vi "Cache User Parameters_minimal_test.vi"(8 "error in (no error)":errorcluster, 11 "SHIFTER DATA in":T1) -> (0 "error out":errorcluster, 3 "SHIFTER DATA out":T1)   [LabVIEW 2013, in "main.lvlib"]
uses:
  Components/TypeDef - SHIFTER.ctl
  Components/Dependencies.llb/Exit Event Ref.ctl
  New Design/Controls/Reference Cluster.ctl
  Controls/Enum Variables.ctl
  main.lvlib
  Components/Dependencies.llb/TLB_Dependencies.lvlib
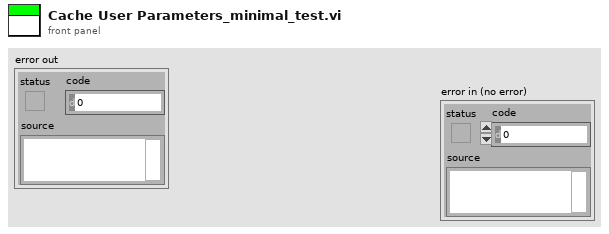
[diagram p1: front panel]
types:
  T1 = typedef "main.lvlib/TypeDef - SHIFTER.ctl" = cluster{"Exit Event":T2, "Terminate Error":errorcluster, "User Parameter Controls":refnum<vi>[], "User Parameters":cluster{"Name":string, "CPR Number":string, "Measuring Type ":string, "Measuring Technique":string, "Measuring Limb":string, "Operator":string, "Doctor":string, "Comment":string, "AdditionalInfo":string, "RightArm":string[][], "LeftArm":string[][], "PalpationRight":string, "PalpationLeft":string, "Puls":dbl, "Temp One":dbl, "Temp Two":dbl, "ActivityBox":bool}, "System Parameters":cluster{"Paper Running?":bool, "GraphSelection":bool, "Date":string, "Active Page":string}, "Data Acquisition":cluster{"Acquisition":bool, "DAQmx Task":refnum<k21>, "DAQmx Error":errorcluster, "Record number":dbl, "RecordPath":path, "AcqDataRef":refnum<vi>, "Duration":timestamp, "Queue":refnum<queue>, "Control?":bool, "RelativeRecordPath":path}, "Reference signal":cluster{"DAQmx  Task ":refnum<k21>, "Monitor":bool, "Events":dbl, "Time":timestamp, "NullEvents":dbl, "RefDataRef":refnum<vi>, "Queue":refnum<queue>}, "Data Process":cluster{"SubpanelRef":refnum<vi>, "ActiveItemTag":string, "Queue":refnum<queue>}, "System Parameter Controls":refnum<vi>[], "Database":cluster{"PatientdataRef":refnum<file>, "PatientdataPath":path, "Blue Pressure":dbl, "Red Pressure":dbl, "ActiveItemTag":string, "Height Adjustment":dbl, "BluePositionArray":dbl[][], "RedPositionArray":dbl[][], "JournalPath":path}, "MWL":cluster{"PatientID":string, "Name":string, "DICOM Info":path, "DICOM Variables":string[], "Worklist":string[][]}, "Control":cluster{"Queue":refnum<queue>, "SignalCluster":cluster{"Pump":bool, "Finger":bool, "Ankle":bool, "Fast Def":bool, "Slow Def":bool, "Init Cal":bool, "Table Pres":bool, "Table":bool}}, "PageMenu":cluster{"VI Reference":refnum<vi>, "Queue":refnum<queue>}, "Profile":cluster{"VI Reference":refnum<vi>, "Queue":refnum<queue>}, "Configuration":cluster{"VI Reference":refnum<vi>, "Queue":refnum<queue>}, "Acquisition":cluster{"VI Reference":refnum<vi>, "Queue":refnum<queue>}, "Data":cluster{"VI Reference":refnum<vi>, "Queue":refnum<queue>}, "Journal":cluster{"VI Reference":refnum<vi>, "Queue":refnum<queue>}, "cRef":T3, "Bluetooth":cluster{"Queue":refnum<queue>, "VI Reference":refnum<vi>}}
  T2 = typedef "main.lvlib/TLB_Dependencies.lvlib/Exit Event Ref.ctl" = refnum<user-event>
  T3 = typedef "main.lvlib/Reference Cluster.ctl" = cluster{"Menu":cluster{"References":cluster{"Stop Acq":refnum<vi>, "MenuExit":refnum<vi>, "MenuStartADC":refnum<vi>, "PersonalInfoString":refnum<vi>, "Profile":refnum<vi>, "Configuration":refnum<vi>, "Acquisition":refnum<vi>, "Data":refnum<vi>, "Journal":refnum<vi>}}, "Profile":cluster{"References":cluster{"Search Patient ID":refnum<vi>, "Name":refnum<vi>, "CommentStr":refnum<vi>, "Listbox Patient ID":refnum<vi>, "ListboxDoctor":refnum<vi>, "ListboxOperator":refnum<vi>, "HospitalName":refnum<vi>, "HospitalDepartment":refnum<vi>, "HospitalAddress":refnum<vi>, "EditHospInfo":refnum<vi>, "Add Patient ID Btn":refnum<vi>, "Query Worklist":refnum<vi>}}, "Configuration":cluster{"References":cluster{"ListboxMeasurementArea":refnum<vi>, "ListboxMeasurementTechnique":refnum<vi>, "ListboxMeasurementMeth":refnum<vi>, "ListboxRightSegmentNr":refnum<vi>, "ListboxLeftSegmentNr":refnum<vi>, "HeightAdjustmentInt":refnum<vi>, "PalpationRight":refnum<vi>, "PalpationLeft":refnum<vi>, "ActivityBox":refnum<vi>}, "New method":cluster{"AddNewMeasurementBtn":refnum<vi>, "Left Time Table":refnum<vi>, "Right Time Table":refnum<vi>}, "Old method":cluster{"LeftArmPressureTable":refnum<vi>, "RightArmPressureTable":refnum<vi>, "SaveArmPressureBtn":refnum<vi>, "Puls":refnum<vi>, "TempTwo":refnum<vi>, "TempOne":refnum<vi>}, "Method":string}, "Acquisition":cluster{"References":cluster{"SegmentAcqString":refnum<vi>, "RingActGraph":refnum<vi>}}, "Data":cluster{"References":cluster{"cmString":refnum<vi>, "AdjustedHeight":refnum<vi>, "Menu":refnum<vi>, "Tangent On/Off":refnum<vi>, "FilterControl":refnum<vi>}}, "Journal":cluster{"References":cluster{"ReportSelection":refnum<vi>, "Data":refnum<vi>, "GenerateReport":refnum<vi>, "Menu":refnum<vi>, "Send To PACS":refnum<vi>}}}
  T4 = typedef "main.lvlib/Enum Variables.ctl" = enum16{"SetAcqFilter", "GetAcqFilter", "Set Filter", "Get Filter", "Set Height", "Get Height", "Set Blue Pressure", "Get Blue Pressure", "Set Red Pressure", "Get Red Pressure", "Init", "Reset Pressure", "Set Red Cursors", "Get Red Cursors", "Set Blue Cursors", "Get Blue Cursors", "Set Language", "Get Language", "Set Active Graphs", "Get ActiveGraphs", "Set Method", "Get Method", "Set Encryption", "Get Encryption", "Set ExcelVersion", "Get ExcelVersion", "Set DICOM Avail", "Get DICOM Avail", "Set DICOM Encode", "Get DICOM Encode", "Set JournalExport", "Get JournalExport", "Set Sequence", "Get Sequence", "Set DAQ Connected", "Get DAQ Connected", "Set Current Graph", "Get Current Graph", "Set General Settings", "Get Hyphenation", "Set Arm Calc Method", "Get Arm Calc Method", "Set Dicom Tags", "Get Dicom Tags", "Set BT Serial", "Get BT Serial", "Set BT Accepted Serials", "Get BT Accepted Serials", "Get BT License", "Set BT License"}
  T5 = cluster{"ListboxMeasurementArea":refnum<vi>, "ListboxMeasurementTechnique":refnum<vi>, "ListboxMeasurementMeth":refnum<vi>, "ListboxRightSegmentNr":refnum<vi>, "ListboxLeftSegmentNr":refnum<vi>, "HeightAdjustmentInt":refnum<vi>, "PalpationRight":refnum<vi>, "PalpationLeft":refnum<vi>, "ActivityBox":refnum<vi>}
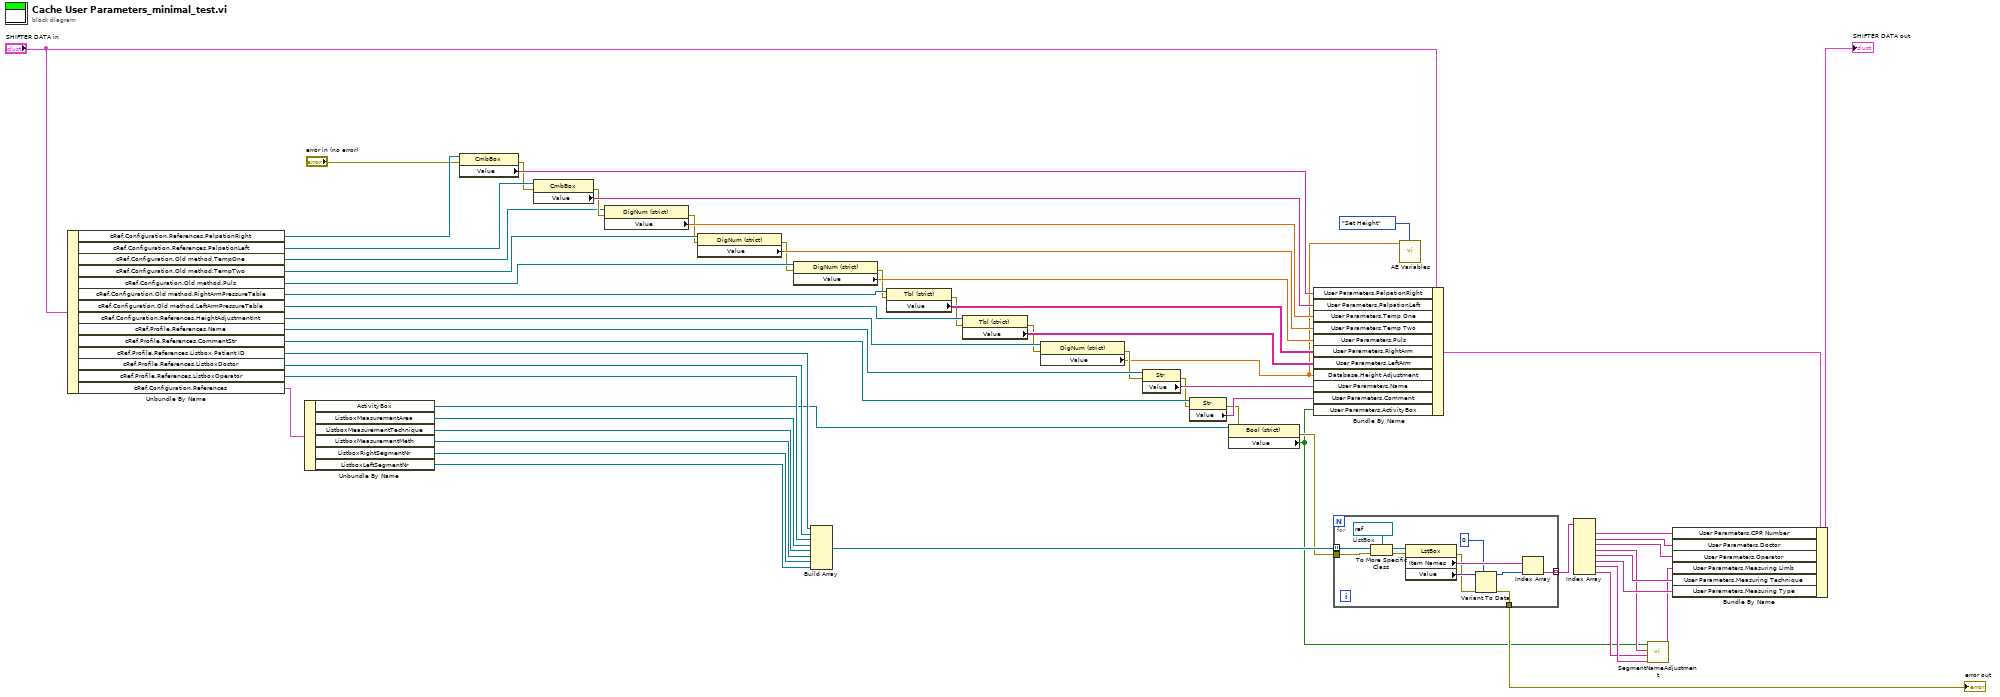
[diagram p0: block diagram]
diagram:
  n1 = Unbundle By Name("SHIFTER DATA in") -> ("cRef.Configuration.References.PalpationRight"=w27:refnum<vi>, "cRef.Configuration.References.PalpationLeft"=w29:refnum<vi>, "cRef.Configuration.Old method.TempOne"=w3:refnum<vi>, "cRef.Configuration.Old method.TempTwo"=w32:refnum<vi>, "cRef.Configuration.Old method.Puls"=w34:refnum<vi>, "cRef.Configuration.Old method.RightArmPressureTable"=w37:refnum<vi>, "cRef.Configuration.Old method.LeftArmPressureTable"=w38:refnum<vi>, "cRef.Configuration.References.HeightAdjustmentInt"=w41:refnum<vi>, "cRef.Profile.References.Name"=w52:refnum<vi>, "cRef.Profile.References.CommentStr"=w51:refnum<vi>, "cRef.Profile.References.Listbox Patient ID"=w15:refnum<vi>, "cRef.Profile.References.ListboxDoctor"=w50:refnum<vi>, "cRef.Profile.References.ListboxOperator"=w49:refnum<vi>, "cRef.Configuration.References"=w11:T5)
  n2 = Unbundle By Name(w11) -> ("ActivityBox"=w5:refnum<vi>, "ListboxMeasurementArea"=w10:refnum<vi>, "ListboxMeasurementTechnique"=w9:refnum<vi>, "ListboxMeasurementMeth"=w8:refnum<vi>, "ListboxRightSegmentNr"=w7:refnum<vi>, "ListboxLeftSegmentNr"=w6:refnum<vi>)
  n3 = property class="CmbBox"(reference=w27, error in="error in (no error)") -> (error out=w25:errorcluster, "Value"=w26:string)  [unwired: 1 out]
  n4 = property class="CmbBox"(reference=w29, error in=w25) -> (error out=w24:errorcluster, "Value"=w28:string)  [unwired: 1 out]
  n5 = property class="DigNum (strict)"(reference=w3, error in=w24) -> (error out=w23:errorcluster, "Value"=w30:dbl)  [unwired: 1 out]
  n6 = property class="DigNum (strict)"(reference=w32, error in=w23) -> (error out=w22:errorcluster, "Value"=w31:dbl)  [unwired: 1 out]
  n7 = property class="DigNum (strict)"(reference=w34, error in=w22) -> (error out=w21:errorcluster, "Value"=w33:dbl)  [unwired: 1 out]
  n8 = Build Array(w15, w50, w49, w10, w9, w8, w7, w6) -> (w54:refnum<vi>[])
  n9 = property class="Tbl (strict)"(reference=w37, error in=w21) -> (error out=w20:errorcluster, "Value"=w35:string[][])  [unwired: 1 out]
  n10 = property class="Tbl (strict)"(reference=w38, error in=w20) -> (error out=w19:errorcluster, "Value"=w36:string[][])  [unwired: 1 out]
  n11 = property class="DigNum (strict)"(reference=w41, error in=w19) -> (error out=w18:errorcluster, "Value"=w1:dbl)  [unwired: 1 out]
  n12 = property class="Str"(reference=w52, error in=w18) -> (error out=w17:errorcluster, "Value"=w39:string)  [unwired: 1 out]
  n13 = property class="Str"(reference=w51, error in=w17) -> (error out=w14:errorcluster, "Value"=w40:string)  [unwired: 1 out]
  n14 = property class="Bool (strict)"(reference=w5, error in=w14) -> (error out=w13:errorcluster, "Value"=w12:bool)  [unwired: 1 out]
  n15 = Bundle By Name(cluster="SHIFTER DATA in", "User Parameters.PalpationRight"=w26, "User Parameters.PalpationLeft"=w28, "User Parameters.Temp One"=w30, "User Parameters.Temp Two"=w31, "User Parameters.Puls"=w33, "User Parameters.RightArm"=w35, "User Parameters.LeftArm"=w36, "Database.Height Adjustment"=w1, "User Parameters.Name"=w39, "User Parameters.Comment"=w40, "User Parameters.ActivityBox"=w12) -> (w44:T1)
  n16 = for {
    tunnel: [w70] -> w55 mode=indexing
    tunnel: w54 -> [w69] mode=indexing
    tunnel: [w60] -> w59
    tunnel: w13 -> [w66]
    w68 = refnum<vi> refnum  # ListBox
    n17 = To More Specific Class(target class=w68, reference=w69, error in=w66) -> (specific class reference=w67:refnum<vi>, error out=w65:errorcluster)
    n18 = property class="LstBox"(reference=w67, error in=w65) -> (error out=w61:errorcluster, "Item Names"=w71:string[], "Value"=w64:variant)  [unwired: 1 out]
    n19 = Variant To Data(error in=w61, type=0, Variant=w64) -> (data=w62:i32, error out=w60:errorcluster)
    n20 = Index Array(array=w71, index=w62) -> (element=w70:string)
  }
  "error out" <- w59
  n21 = call "AE Variables.vi"("VariantIn"=w1, "Action"=Enum_Variables."Set Height") -> ()  [unwired: 10 in, 8 out]
  n22 = Index Array(array=w55) -> (element #1=w56:string, element #2=w43:string, element #3=w42:string, element #4=w48:string, element #5=w57:string, element #6=w58:string, element #7=w47:string, element #8=w46:string)  [unwired: 8 in]
  n23 = call "SegmentNameAdjustment.vi"("Right"=w47, "Left"=w46, "Segment In"=w48, "Activity"=w12) -> ("Segment Out"=w45:string)  [unwired: 7 in]
  n24 = Bundle By Name(cluster=w44, "User Parameters.CPR Number"=w56, "User Parameters.Doctor"=w43, "User Parameters.Operator"=w42, "User Parameters.Measuring Limb"=w45, "User Parameters.Measuring Technique"=w57, "User Parameters.Measuring Type"=w58) -> (→"SHIFTER DATA out":T1)
